vi "彩色直方图2.vi"() -> ()   [LabVIEW 2018]
uses:
  <vilib>/vision/NI_Vision_Development_Module.lvlib
panel:
  out "error out":errorcluster
  out "波形图 3":T1(graph)
  out "波形图 2":T1(graph)
  out "波形图":T1(graph)
  out "Image":T2(plugin-control)
  in  "路径":path
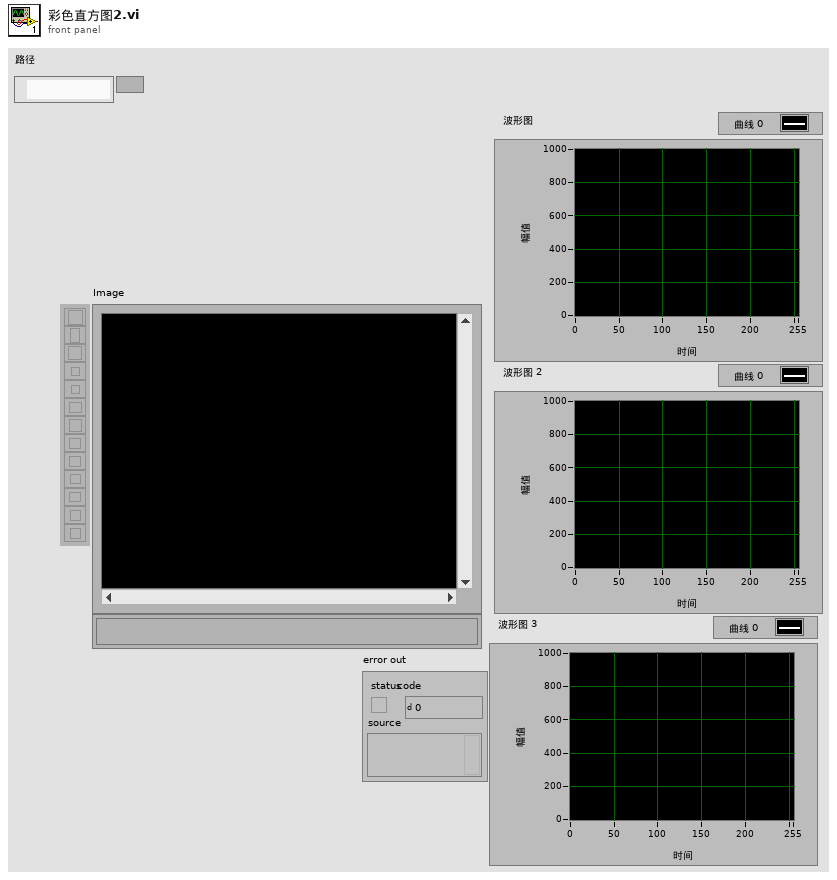
[diagram p1: front panel]
types:
  T1 = cluster{"Starting Value":sgl, "Incremental Value":sgl, "Histogram":u32[]}
  T2 = typedef "IMAQ Image.ctl" = refnum<image>
  T3 = typedef "Image Type" = u32
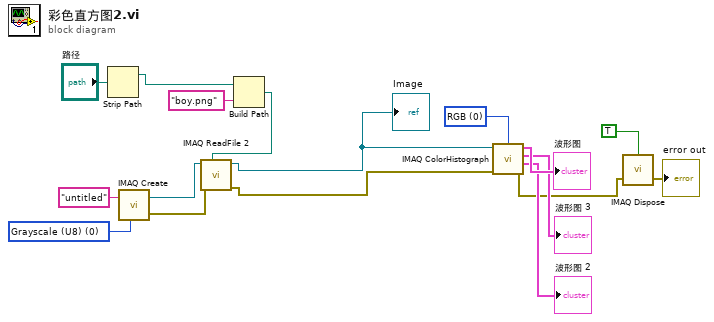
[diagram p0: block diagram]
diagram:
  w9 = u16 0 items=["RGB", "HSL", "HSV", "HSI"] ("Color Mode")
  w13 = T3 0 items=["Grayscale (U8)", "Grayscale (I16)", "Grayscale (SGL)", "Complex (CSG)", "RGB (U32)", "HSL (U32)", "RGB (U64)", "Grayscale (U16)"] ("Image Type")
  n1 = Strip Path(path="路径") -> (stripped path=w16:path)  [unwired: 1 out]
  n2 = call "IMAQ Create"("Image Name"="untitled", "Image Type"=w13) -> ("New Image"=w12:T2, "error out"=w11:errorcluster)  [unwired: 3 in]
  n3 = Build Path(base path=w16, name or relative path="boy.png" ("名称或相对路径")) -> (appended path=w15:path)
  n4 = call "IMAQ ReadFile 2"("File Path"=w15, "error in (no error)"=w11, "Image"=w12) -> ("error out"=w2:errorcluster, "Image Out"=w1:T2)  [unwired: 4 in, 3 out]
  "Image" <- w1
  n5 = call "IMAQ ColorHistograph"("Color Mode"=w9, "Image Src"=w1, "error in (no error)"=w2) -> ("Red or Hue Histogram Graph"=→"波形图":T1, "Green or Sat Histogram Graph"=→"波形图 3":T1, "Blue or Luma or Val or Inten Histogram Graph"=→"波形图 2":T1, "error out"=w5:errorcluster)  [unwired: 3 in]
  n6 = call "IMAQ Dispose"("All Images? (No)"=TRUE, "error in (no error)"=w5) -> ("error out"=→"error out":errorcluster)  [unwired: 4 in]
